vi "MSEncoder SubVI Beta2Q.vi"(10 "Beta":dbl) -> (2 "Q":dbl)   [LabVIEW 2018]
uses:
  <vilib>/Analysis/NI_AALPro.lvlib
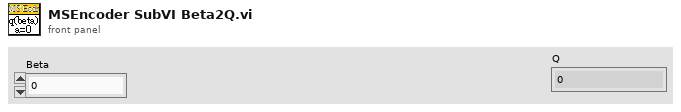
[diagram p1: front panel]
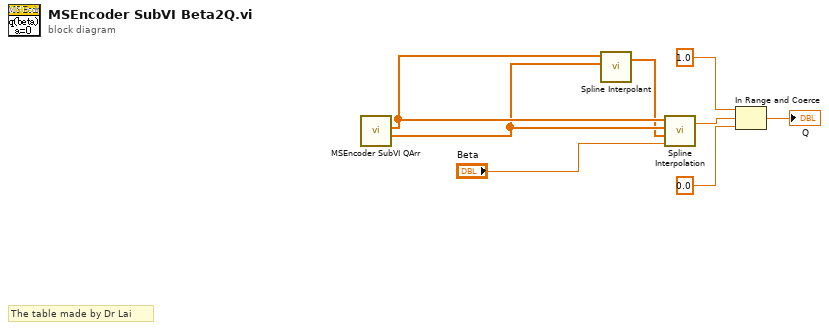
[diagram p0: block diagram]
diagram:
  # "The table made by Dr Lai"
  n1 = call "MSEncoder SubVI QArr.vi"() -> ("Beta"=w5:dbl[], "Q"=w8:dbl[])  [unwired: 10 in]
  n2 = call <vilib>:"Spline Interpolant.vi"("X"=w5, "Y"=w8) -> ("Interpolant"=w1:dbl[])  [unwired: 2 in, 1 out]
  n3 = call <vilib>:"Spline Interpolation.vi"("x value"="Beta", "Interpolant"=w1, "X"=w5, "Y"=w8) -> ("interpolation value"=w6:dbl)  [unwired: 1 out]
  n4 = In Range and Coerce(upper limit=1.0, x=w6, lower limit=0.0) -> (coerced(x)=→"Q":dbl)  [unwired: 1 out]
